vi "sq_controller.vi"(4 "Degraded":bool[](array[boolean]), 6 "Reset":bool, 7 "Parameters":T1={"Stimulus"={"Type"=enum."Off", "Phase"=0.0, "Amplitude"=[], "Injection point"=enum."Total pose", "Closed loop"=FALSE, "Offset"=[], "Tip -> world"=FALSE, "Frequency"=0.0, "Length"=0.0}, "Goal Filter A"={"Speedup max"=0.0, "Speedup thresh"=0.0, "Speedup nonlin"=0.0, "Filters"=[]}, "Mode controls"={"Hold"=FALSE, "Cancellation"=FALSE, "Goal filter"=FALSE, "Trigger"=FALSE}, "Manipulator type"=enum."Current piezo", "Manipulator calibration"={"Tool offsets"=[[0.0, 0.0, 36200.0]], "Tip light calibration"=[], "Handle light calibration"=[], "Base pivots"=[], "Output pivots"=[], "Length center"=0.0, "Workspace height"=[], "Workspace diameter"=[0.0, 0.0, 36200.0], "Linearization"=[[0.0, 0.0, 36200.0]], "Stack travel"=400.0, "Saturation pos"=375.0, "Inverse filters"=[]}, "Network"={"Remote Host"="", "Send Status"=FALSE, "Send Port"=0, "Recv Commands"=FALSE, "Recv Port"=0}, "Goal Filter B"={"Speedup max"=0.0, "Speedup thresh"=0.0, "Speedup nonlin"=0.0, "Filters"=[]}, "Cancellation"={"KP"={"XY"=0.0, "Rxy"=0.0, "Z"=0.0, "Rz"=0.0}, "KI"=0.0, "KD"={"XY"=0.0, "Rxy"=0.0, "Z"=0.0, "Rz"=0.0}, "Max vel"=20.0, "Max acc"=0.001, "Int error limit"=3.0, "RCM gain"=0.0, "Bypass"=FALSE, "Degraded gain"=0.0}, "Transition time"=0.0, "Estimation"={"Link"={"Measure noise"=[], "Process noise"=[], "Alt process noise"=[], "Alt turnoff cycles"=20, "Innovation limit"=[], "Residue threshold"=0.0, "Enable"=FALSE}, "Handle"={"Measure noise"=[], "Process noise"=[], "State limits"=[], "Innovation limit"=[], "Prediction Lookahead"=0.0, "Enable"=FALSE}}} {"Transition time" format="%_3f"; "Cancellation"."Degraded gain" min=0 max=1 step=0.1 format="%#_3p"; "Cancellation"."RCM gain" min=0 max=1 step=0.1 format="%#_3p"; "Cancellation"."KD"."Rz" min=0 max=1 step=0.1 format="%#_3p"; "Cancellation"."KD"."Rxy" min=0 max=1 step=0.1 format="%#_3p"; "Cancellation"."KD"."Z" min=0 max=1 step=0.1 format="%#_3p"; "Cancellation"."KD"."XY" min=0 max=1 step=0.1 format="%#_3p"; "Cancellation"."KI" min=0 max=1 step=0.01 format="%#_3p"; "Cancellation"."KP"."Rz" min=0 max=1 step=0.1 format="%#_3p"; "Cancellation"."KP"."Rxy" min=0 max=1 step=0.1 format="%#_3p"; "Cancellation"."KP"."Z" min=0 max=1 step=0.1 format="%#_3p"; "Cancellation"."KP"."XY" min=0 max=1 step=0.1 format="%#_3p"; "Cancellation"."Max acc" format="%#_3p"; "Goal Filter B"."Filters"."V limit range" format="%_3p"; "Goal Filter B"."Filters"."V limit" format="%_3p"; "Goal Filter B"."Filters"."Upper Q" format="%_3f"; "Goal Filter B"."Filters"."Upper Fc" format="%_3p"; "Goal Filter B"."Filters"."Lower Q" format="%_3f"; "Goal Filter B"."Filters"."Scale factor" format="%_3f"; "Goal Filter B"."Filters"."Lower Fc" format="%_3p"; "Goal Filter B"."Speedup nonlin" format="%_3p"; "Goal Filter B"."Speedup thresh" format="%_3p"; "Goal Filter B"."Speedup max" format="%_3p"; "Manipulator calibration"."Saturation pos" format="%#.1f"; "Manipulator calibration"."Stack travel" format="%#.1f"; "Manipulator calibration"."Output pivots" format="%#_6f"; "Manipulator calibration"."Base pivots" format="%#_6f"; "Manipulator calibration"."Handle light calibration" format="%#.1f"; "Manipulator calibration"."Tip light calibration" format="%#.1f"; "Goal Filter A"."Filters"."V limit range" format="%_3p"; "Goal Filter A"."Filters"."V limit" format="%_3p"; "Goal Filter A"."Filters"."Upper Q" format="%_3f"; "Goal Filter A"."Filters"."Upper Fc" format="%_3p"; "Goal Filter A"."Filters"."Lower Q" format="%_3f"; "Goal Filter A"."Filters"."Scale factor" format="%_3f"; "Goal Filter A"."Filters"."Lower Fc" format="%_3p"; "Goal Filter A"."Speedup nonlin" format="%_3p"; "Goal Filter A"."Speedup thresh" format="%_3p"; "Goal Filter A"."Speedup max" format="%_3p"; "Stimulus"."Length" min=0.0 max=100.0 step=100.0 format="%#_4p"; "Stimulus"."Frequency" min=0.0 step=100.0 format="%#_4g"; "Stimulus"."Offset" format="%#_3p"; "Stimulus"."Amplitude" format="%#_3p"; "Stimulus"."Phase" min=-180.0 max=360.0 step=100.0 format="%#.2f"}, 8 "Link rates":sgl[](array[numeric]), 10 "Link length error":sgl[](array[numeric])) -> (5 "Motor commands":sgl[](array[numeric]))   [LabVIEW 2013]
uses:
  testing/Micron params.ctl
  testing/stimulus.ctl
  testing/injection_point.ctl
  filtering/goal_loop_parms.ctl
  testing/mode_conrols.ctl
  testing/manipulator_cal.ctl
  asap/labview/testing/probe_calibration.ctl
  host/network_params.ctl
  sq_control_params.ctl
  decoupled_gain.ctl
  estimation_controls.ctl
  calibration/dynamic_mode.ctl
panel:
  in  "Integral error":sgl[](array[numeric])=[0.0, 0.0, 0.0, 0.0, 0.0, 0.0]
  # "Integral error term has saturated (stall condition)"
  # "Locals:"
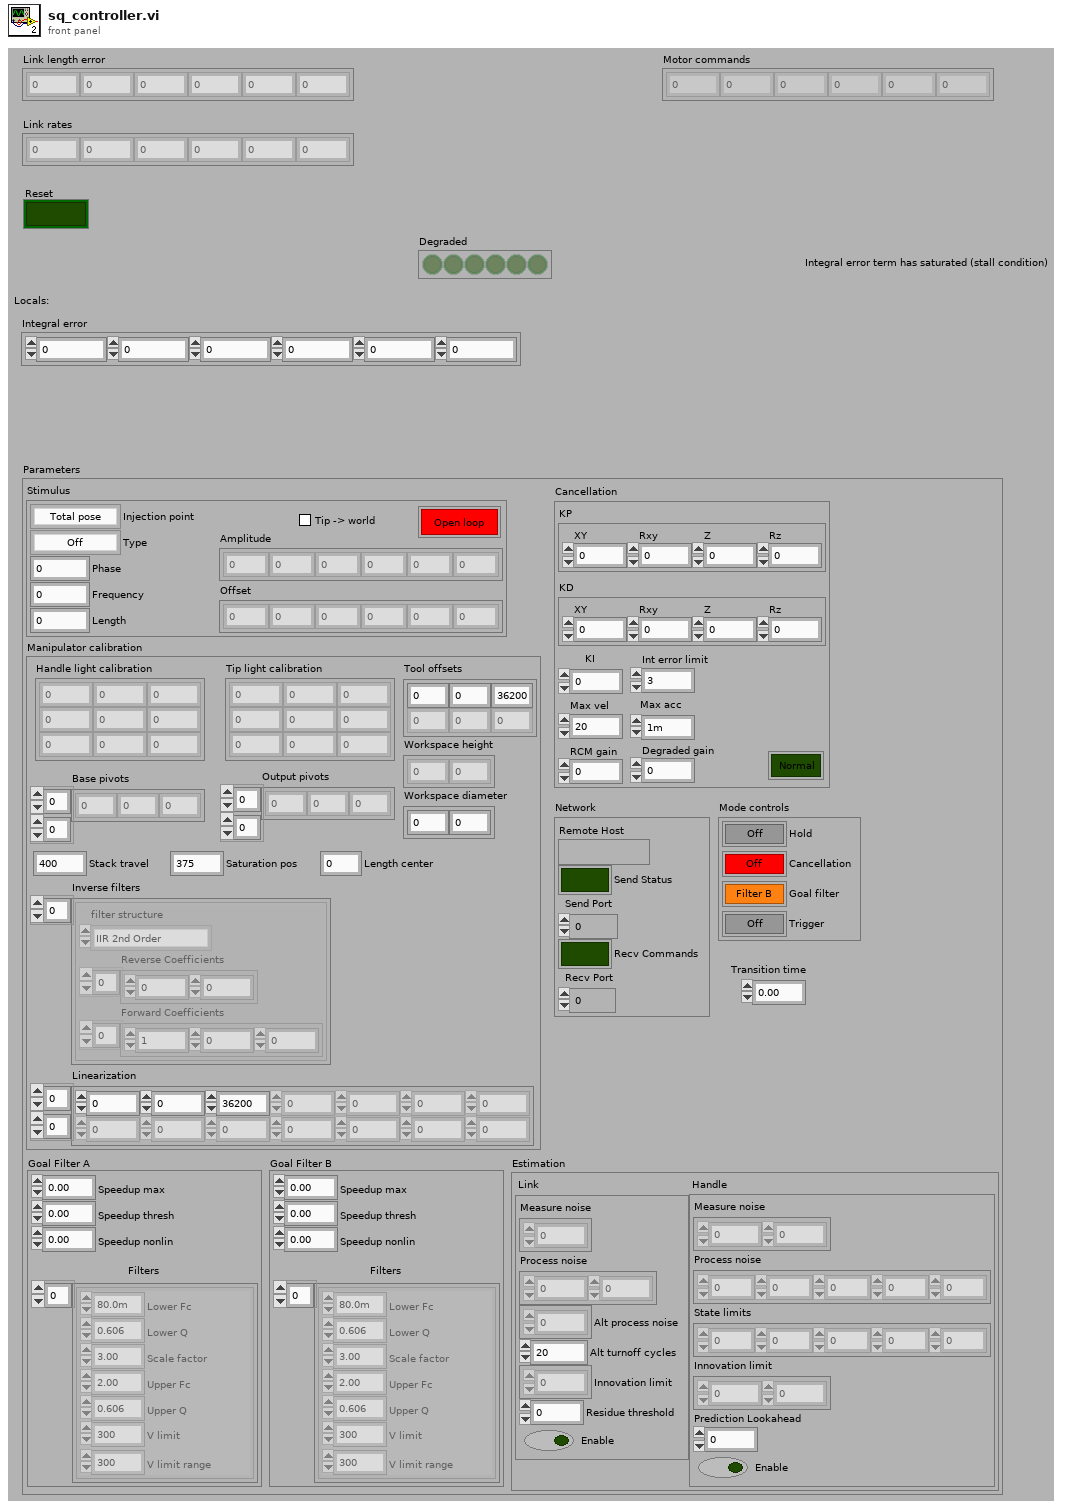
[diagram p1: front panel]
types:
  T1 = typedef "Micron params.ctl" = cluster{"Stimulus":T2, "Goal Filter A":T4, "Mode controls":T5, "Manipulator type":enum16{"Current piezo", "Voltage piezo"}, "Manipulator calibration":T6, "Network":T8, "Goal Filter B":T4, "Cancellation":T9, "Transition time":sgl, "Estimation":T11}
  T2 = typedef "stimulus.ctl" = cluster{"Type":enum16{"Off", "Step", "Sine", "Triangle", "Arbitrary"}, "Phase":dbl, "Amplitude":sgl[], "Injection point":T3, "Closed loop":bool, "Offset":sgl[], "Tip -> world":bool, "Frequency":dbl, "Length":dbl}
  T3 = typedef "injection_point.ctl" = enum16{"Total pose", "V limiter", "Goal ", "Link position", "KF link position", "Inverse kin", "Link goal", "Link error", "Controller", "Output", "Drive", "Light"}
  T4 = typedef "goal_loop_parms.ctl" = cluster{"Speedup max":sgl, "Speedup thresh":sgl, "Speedup nonlin":sgl, "Filters":cluster{"Lower Fc":sgl, "Lower Q":sgl, "Scale factor":sgl, "Upper Fc":sgl, "Upper Q":sgl, "V limit":sgl, "V limit range":sgl}[]}
  T5 = typedef "mode_conrols.ctl" = cluster{"Hold":bool, "Cancellation":bool, "Goal filter":bool, "Trigger":bool}
  T6 = typedef "manipulator_cal.ctl" = cluster{"Tool offsets":sgl[][], "Tip light calibration":T7, "Handle light calibration":T7, "Base pivots":sgl[][], "Output pivots":sgl[][], "Length center":sgl, "Workspace height":sgl[], "Workspace diameter":sgl[], "Linearization":sgl[][], "Stack travel":sgl, "Saturation pos":sgl, "Inverse filters":cluster{"filter structure":enum32{"IIR 2nd Order", "IIR 4th Order"}, "Reverse Coefficients":dbl[], "Forward Coefficients":dbl[]}[]}
  T7 = typedef "probe_calibration.ctl" = sgl[][]
  T8 = typedef "network_params.ctl" = cluster{"Remote Host":string, "Send Status":bool, "Send Port":u16, "Recv Commands":bool, "Recv Port":u16}
  T9 = typedef "sq_control_params.ctl" = cluster{"KP":T10, "KI":sgl, "KD":T10, "Max vel":sgl, "Max acc":sgl, "Int error limit":sgl, "RCM gain":sgl, "Bypass":bool, "Degraded gain":sgl}
  T10 = typedef "decoupled_gain.ctl" = cluster{"XY":sgl, "Rxy":sgl, "Z":sgl, "Rz":sgl}
  T11 = typedef "estimation_controls.ctl" = cluster{"Link":cluster{"Measure noise":dbl[], "Process noise":dbl[], "Alt process noise":dbl[], "Alt turnoff cycles":i32, "Innovation limit":dbl[], "Residue threshold":dbl, "Enable":bool}, "Handle":cluster{"Measure noise":dbl[], "Process noise":dbl[], "State limits":dbl[], "Innovation limit":dbl[], "Prediction Lookahead":sgl, "Enable":bool}}
  T12 = typedef "dynamic_mode.ctl" = enum16{"XY", "Rxy", "Z", "Rz"}
  T13 = cluster{"filter structure":enum32{"IIR 2nd Order", "IIR 4th Order"}, "Reverse Coefficients":dbl[], "Forward Coefficients":dbl[]}[]
  T14 = cluster{"filter structure":enum32{"IIR 2nd Order", "IIR 4th Order"}, "Reverse Coefficients":dbl[], "Forward Coefficients":dbl[]}
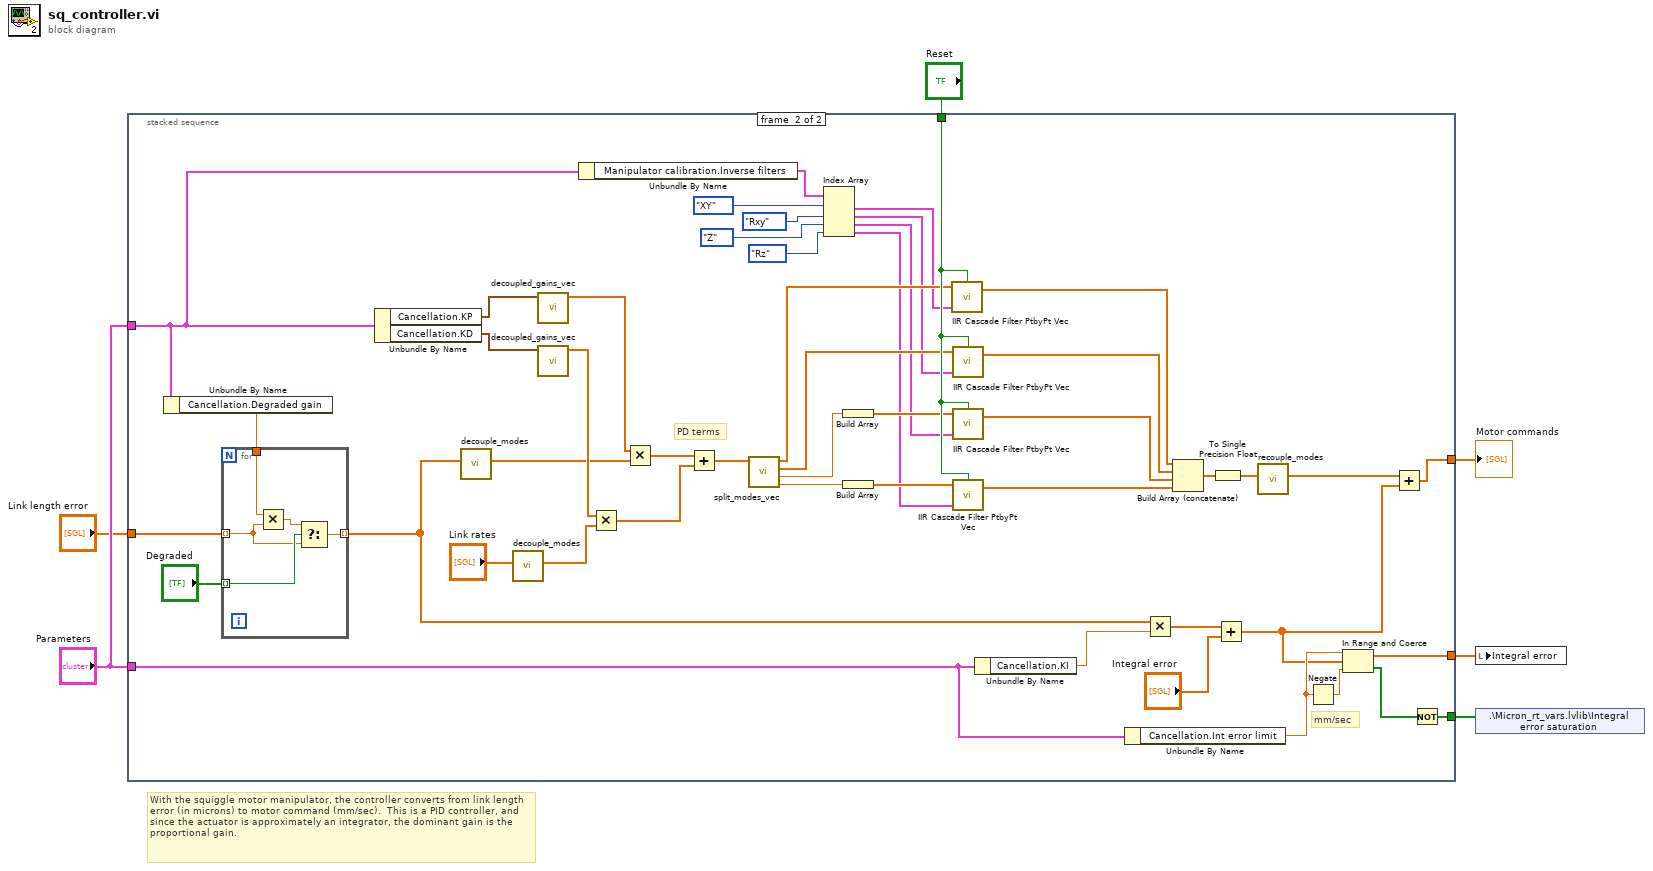
[diagram p0: block diagram]
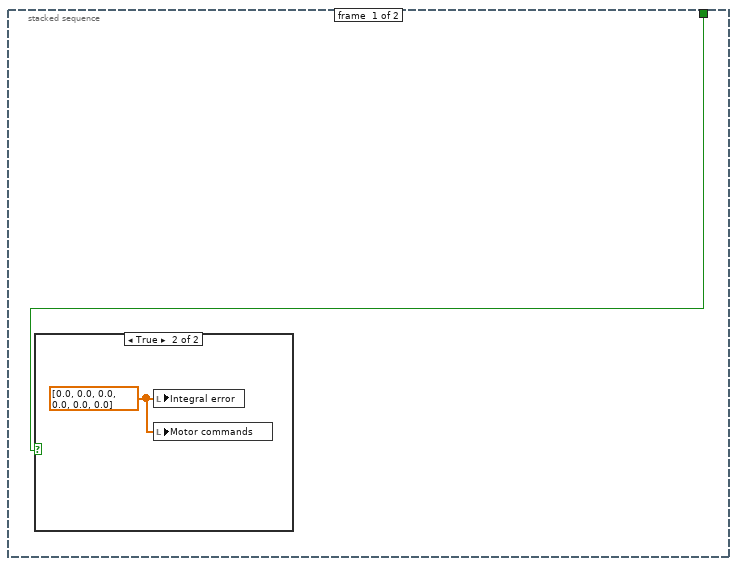
[diagram p2: hidden frame]
diagram:
  # "With the squiggle motor manipulator, the controller converts from link length error (in microns) to motor command (mm/sec).  This is a PID controller, and since the actuator is approximately an integrator, the dominant gain is the proportional gain."
  n1 = stacked-sequence {
    tunnel: "Link length error" -> [_ w13]
    tunnel: "Parameters" -> [_ w50]
    tunnel: "Parameters" -> [_ w10]
    tunnel: [_ w53] -> w4
    tunnel: [_ w47] -> w1
    tunnel: [_ w46] -> w3
    tunnel: "Reset" -> [w7 w36]
    frame #0 {
      n2 = case shown="True" w7 {
        frame False {
        }
        frame True {
          w8 = sgl[] [0.0, 0.0, 0.0, 0.0, 0.0, 0.0] ("Integral error")
          n3 = local write "Integral error"(w8) -> ()
          n4 = local write "Motor commands"(w8) -> ()
        }
      }
    }
    frame #1 {
      # "mm/sec"
      # "PD terms"
      n5 = Unbundle By Name(w10) -> ("Cancellation.Degraded gain"=w9:sgl)
      n6 = for {
        tunnel: w13 -> [w59] mode=indexing
        tunnel: [w58] -> w12 mode=indexing
        tunnel: "Degraded" -> [w62] mode=indexing
        tunnel: w9 -> [w60]
        n7 = Multiply(x=w60, y=w59) -> (x*y=w61:sgl)
        n8 = Select(t=w61, s=w62, f=w59) -> (s? t:f=w58:sgl)
      }
      n9 = Unbundle By Name(w10) -> ("Cancellation.KP"=w45:T10, "Cancellation.KD"=w42:T10)
      n10 = call "decouple_modes.vi"("Input"=w12) -> ("Decoupled"=w39:sgl[])  [unwired: 10 in]
      n11 = call "decouple_modes.vi"("Input"="Link rates") -> ("Decoupled"=w40:sgl[])  [unwired: 10 in]
      n12 = call "decoupled_gains_vec.vi"("Gain"=w45) -> ("Decoupled"=w44:sgl[])  [unwired: 10 in]
      n13 = call "decoupled_gains_vec.vi"("Gain"=w42) -> ("Decoupled"=w41:sgl[])  [unwired: 10 in]
      n14 = Unbundle By Name(w10) -> ("Manipulator calibration.Inverse filters"=w29:T13)
      n15 = Multiply(x=w41, y=w40) -> (x*y=w56:sgl[])
      n16 = Multiply(x=w44, y=w39) -> (x*y=w57:sgl[])
      n17 = Add(x=w57, y=w56) -> (x+y=w37:sgl[])
      n18 = call "split_modes_vec.vi"("Decoupled"=w37) -> ("Rz"=w31:sgl, "Z"=w33:sgl, "Rx Ry"=w34:sgl[], "XY"=w35:sgl[])  [unwired: 7 in]
      n19 = Index Array(array=w29, index #1=dynamic_mode."XY" ("Dynamic mode"), index #2=dynamic_mode."Rxy" ("Dynamic mode"), index #3=dynamic_mode."Z" ("Dynamic mode"), index #4=dynamic_mode."Rz" ("Dynamic mode")) -> (element #1=w28:T14, element #2=w27:T14, element #3=w26:T14, element #4=w25:T14)
      n20 = Build Array(w33) -> (w32:sgl[])
      n21 = Build Array(w31) -> (w30:sgl[])
      n22 = call "IIR Cascade Filter PtbyPt Vec.vi"("initialize"=w36, "IIR Filter Cluster"=w28, "X"=w35) -> ("Filtered X"=w24:dbl[])  [unwired: 1 in, 1 out]
      n23 = call "IIR Cascade Filter PtbyPt Vec.vi"("initialize"=w36, "IIR Filter Cluster"=w27, "X"=w34) -> ("Filtered X"=w23:dbl[])  [unwired: 1 in, 1 out]
      n24 = call "IIR Cascade Filter PtbyPt Vec.vi"("initialize"=w36, "IIR Filter Cluster"=w26, "X"=w32) -> ("Filtered X"=w22:dbl[])  [unwired: 1 in, 1 out]
      n25 = call "IIR Cascade Filter PtbyPt Vec.vi"("initialize"=w36, "IIR Filter Cluster"=w25, "X"=w30) -> ("Filtered X"=w21:dbl[])  [unwired: 1 in, 1 out]
      n26 = Unbundle By Name(w50) -> ("Cancellation.KI"=w54:sgl)
      n27 = Unbundle By Name(w50) -> ("Cancellation.Int error limit"=w49:sgl)
      n28 = Multiply(x=w12, y=w54) -> (x*y=w52:sgl[])
      n29 = Build Array (concatenate)(w24, w23, w22, w21) -> (w20:dbl[])
      n30 = To Single Precision Float(number=w20) -> (single precision float=w19:sgl[])
      n31 = Add(x=w52, y="Integral error") -> (x+y=w38:sgl[])
      n32 = call "recouple_modes.vi"("Decoupled"=w19) -> ("Output"=w18:sgl[])  [unwired: 10 in]
      n33 = Negate(x=w49) -> (-x=w51:sgl)
      n34 = In Range and Coerce(upper limit=w49, x=w38, lower limit=w51) -> (coerced(x)=w53:sgl[], In Range?=w48:bool[])
      n35 = Add(x=w18, y=w38) -> (x+y=w46:sgl[])
      n36 = Not(x=w48) -> (.not. x?=w47:bool[])
    }
  }
  "Motor commands" <- w3
  n37 = local write "Integral error"(w4) -> ()
  n38 = shared-variable ".\\Micron_rt_vars.lvlib\\Integral error saturation"(w1) -> ()  [unwired: 2 out]
